vi "三角波形.vi"() -> ()   [LabVIEW 2010]
uses:
  <vilib>/measure/NI_MABase.lvlib
panel:
  in  "等待时间（毫秒）":u32
  in  "phase":dbl caption="相位" format="%.2p"
  in  "amplitude":dbl=1.0 caption="幅值" format="%0.2p"
  in  "frequency":dbl=10.0 caption="频率" format="%0.2p"
  in  "offset":dbl caption="偏移量" format="%0.2p"
  out "Y":dbl[](array[numeric])
  out "dt":dbl
  in  "停止":bool
  in  "sampling info":cluster{"Fs":dbl, "#s":dbl}={"Fs"=1000.0, "#s"=1000.0} caption="采样信息" {"Fs" format="%.2p"}
  out "波形图表":waveform(dbl)(graph)
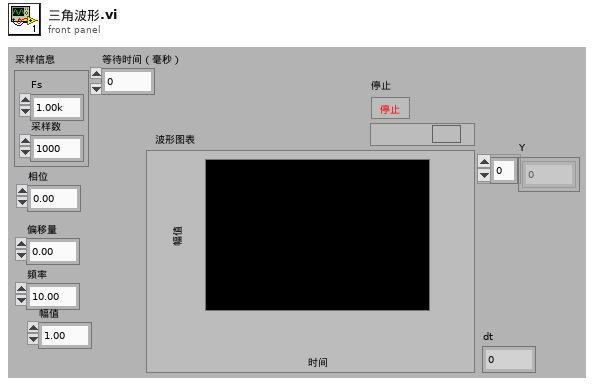
[diagram p1: front panel]
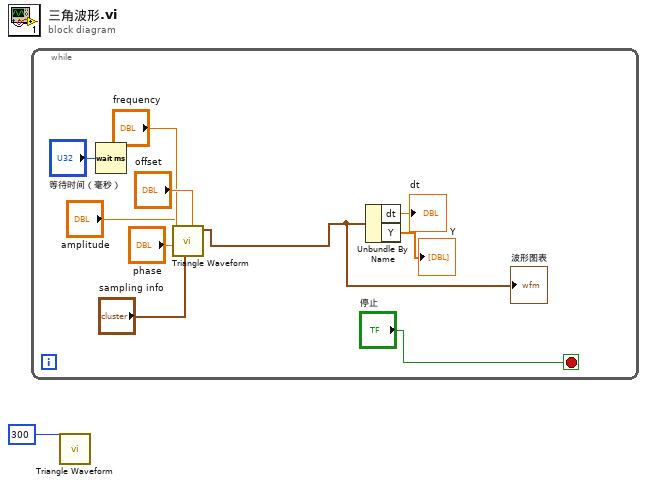
[diagram p0: block diagram]
diagram:
  n1 = while {
    stop <- "停止" stop-if-true
    n2 = Wait (ms)(milliseconds to wait="等待时间（毫秒）") -> ()  [unwired: 1 out]
    n3 = call <vilib>:"Triangle Waveform.vi"("offset"="offset", "sampling info"="sampling info", "phase"="phase", "amplitude"="amplitude", "frequency"="frequency") -> ("signal out"=w7:waveform(dbl))  [unwired: 5 in, 1 out]
    "波形图表" <- w7
    n4 = Unbundle By Name(w7) -> ("dt"=→"dt":dbl, "Y"=→"Y":dbl[])
  }
  n5 = call <vilib>:"Triangle Waveform.vi"("frequency"=300) -> ()  [unwired: 9 in, 2 out]
